vi "Filter Dialog.vi"() -> (0 "error out":errorcluster, 2 "Base Filter out":refnum<class "Base Filter.lvclass">, 3 "Valid Filter Configuration":bool)   [LabVIEW 2018, in "Assert API Components.lvlib" / "Assert Display.lvlib" / "Filter Config Display.lvlib" / "Filter Config Display.lvclass"]
doc: "Filter definition window - allows the user to create new filters on the fly to display/not display assert values in the UI"
uses:
  Filter Config Display.lvclass
  Assert API Components/Filter Type.ctl
  Assert API Components/Filter By Time.ctl
  Assert API Components/Filter By String.ctl
  Assert API Components/Filter Configurations/Base Filter.lvclass
  Assert API Components/Boolean Filter Configuration.ctl
  Assert API Components/Time Filter Configuration.ctl
  Assert API Components/String Filter Configuration.ctl
  Assert API Components/Filter Configurations/Base Filter.lvclass/Base Filter.ctl
  <vilib>/Utility/config.llb/Read Key (String).vi
  Assert Display/Assert Display.lvlib
  Assert API Components/Assert API Components.lvlib
  <vilib>/Utility/config.llb/NI_LVConfig.lvlib
panel:
  in  "Tab Control":enum32{"Boolean", "String", "Time"}(tab)
  in  "Status":bool
  in  "Filter String":T1
  in  "String Comparison Method":T2(ring)
  in  "Filter Value":string
  in  "Filter Time":T3
  in  "Time Comparison Method":enum16{"Before", "After"}(ring)
  in  "Filter Timestamp":timestamp
  in  "Include or Exclude":enum16{"Include", "Exclude"}(ring)
  in  "Filter Type":T4
  in  "OK Button":bool
  in  "Description":string
  in  "Filter Name":string
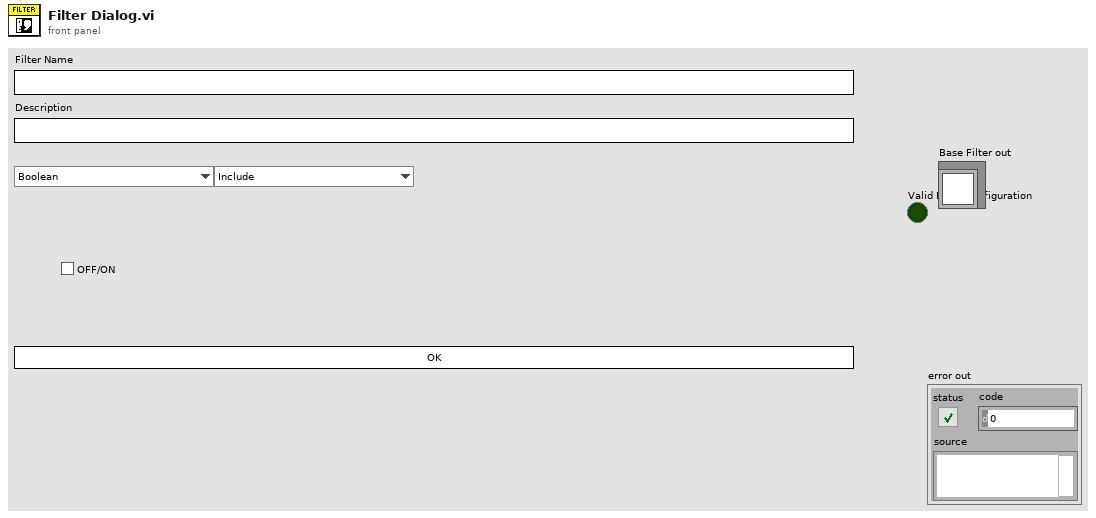
[diagram p1: front panel]
types:
  T1 = typedef "Assert API Components.lvlib/Assert Display.lvlib/Filter By String.ctl" = enum16{"Assert Builder User Name", "Assert Name", "Assert VI Name", "Calling VI Name", "Comment", "Data Type", "Evaluation String"}
  T2 = enum16{"Contains", "Does Not Contain", "Starts With", "Equals", "Does Not Equal"}
  T3 = typedef "Assert API Components.lvlib/Assert Display.lvlib/Filter By Time.ctl" = enum16{"Assert Build Timestamp", "Last Update Timestamp"}
  T4 = typedef "Assert API Components.lvlib/Assert Display.lvlib/Filter Type.ctl" = enum16{"Boolean", "String", "Time"}
  T5 = typedef "Assert API Components.lvlib/Assert Display.lvlib/String Filter Configuration.ctl" = cluster{"Filter String":T1, "String Comparison Method":enum16{"Contains", "Does Not Contain", "Starts With", "Equals", "Does Not Equal"}, "Comparison Value":string}
  T6 = typedef "Assert API Components.lvlib/Assert Display.lvlib/Time Filter Configuration.ctl" = cluster{"Filter Time":T3, "Time Comparison Method":enum16{"Before", "After"}, "Time Stamp":timestamp}
  T7 = typedef "Assert API Components.lvlib/Assert Display.lvlib/Boolean Filter Configuration.ctl" = cluster{"Boolean Comparison Value":bool}
  T8 = typedef "NI_LVConfig.lvlib/Config Data RefNum.ctl" = refnum<k1>
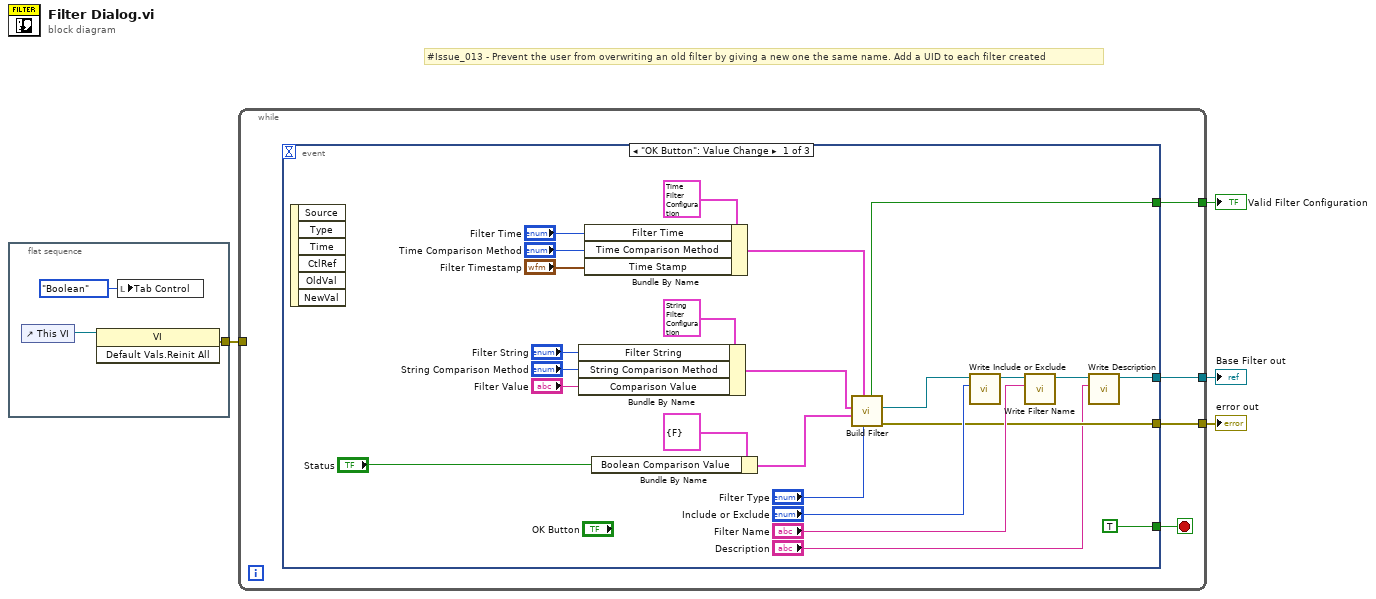
[diagram p0: block diagram]
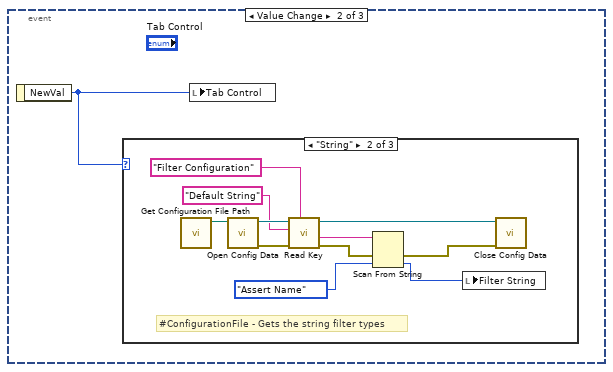
[diagram p2: hidden frame]
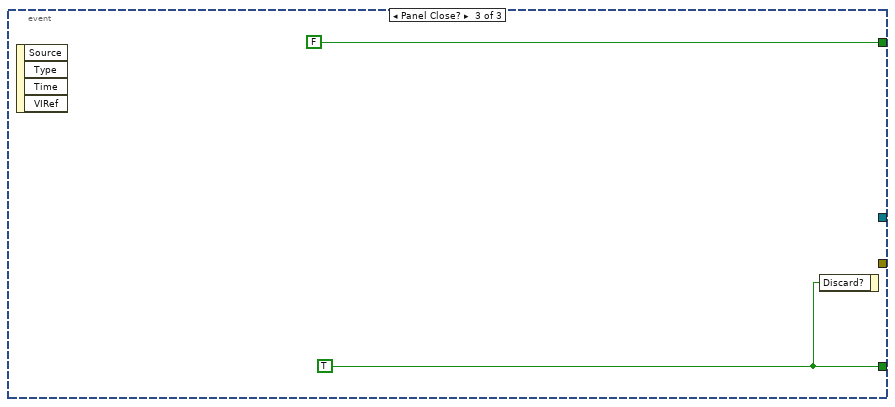
[diagram p5: hidden frame]
diagram:
  # "#Issue_013 - Prevent the user from overwriting an old filter by giving a new one the same name. Add a UID to each filter created"
  n1 = flat-sequence {
    tunnel: [w5] -> w1
    frame #0 {
      n2 = control-ref of="This VI"() -> (w6:refnum<vi>)
      n3 = invoke class="VI" method="Default Vals.Reinit All"(reference=w6) -> (error out=w5:errorcluster)  [unwired: 2 in, 2 out]
      n4 = local write "Tab Control"(enum32{"Boolean", "String", "Time"}."Boolean" ("Tab Control")) -> ()
    }
  }
  n5 = while {
    tunnel: [w10] -> w4
    tunnel: [w9] -> w3
    tunnel: [w8] -> w2
    tunnel: w1 -> [_]
    stop <- w11 stop-if-true
    n6 = event shown="[0] \"OK Button\": Value Change" {
      selector: _ -> [_ _ _]
      dyn-events: _ -> [_ _ _]
      timeout: _ -> [_ _ _]
      tunnel: [TRUE _ w49] -> w11
      tunnel: [w21 _ FALSE] -> w10
      tunnel: [w13 _ _] -> w9
      tunnel: [w14 _ _] -> w8
      event "OK Button": Value Change {
        n7 = event-data() -> ()  [unwired: 1 in, 6 out]
        n8 = Bundle By Name(cluster=T5 {"Filter String"=enum."Assert Builder User Name", "String Comparison Method"=enum."Contains", "Comparison Value"=""}, "Filter String"="Filter String", "String Comparison Method"="String Comparison Method", "Comparison Value"="Filter Value") -> (w29:T5)
        n9 = Bundle By Name(cluster=T6 {"Filter Time"=enum."Assert Build Timestamp", "Time Comparison Method"=enum."Before", "Time Stamp"=timestamp(0 s since 1904-01-01)}, "Filter Time"="Filter Time", "Time Comparison Method"="Time Comparison Method", "Time Stamp"="Filter Timestamp") -> (w27:T6)
        n10 = Bundle By Name(cluster=T7 {"Boolean Comparison Value"=FALSE}, "Boolean Comparison Value"="Status") -> (w28:T7)
        n11 = call "Build Filter.vi"("Filter Type"="Filter Type", "Time Filter Configuration"=w27, "Boolean Filter Configuration"=w28, "String Filter Configuration"=w29) -> ("error out"=w14:errorcluster, "Base Filter out"=w31:refnum<class "Base Filter.lvclass">, "Boolean"=w21:bool)  [unwired: 5 in]
        n12 = call "Write Include or Exclude.vi"("Include or Exclude"="Include or Exclude", "Base Filter in"=w31) -> ("Base Filter out"=w34:refnum<class "Base Filter.lvclass">)  [unwired: 9 in]
        n13 = call "Write Filter Name.vi"("Filter Name"="Filter Name", "Base Filter in"=w34) -> ("Base Filter out"=w15:refnum<class "Base Filter.lvclass">)  [unwired: 9 in]
        n14 = call "Write Description.vi"("Description"="Description", "Base Filter in"=w15) -> ("Base Filter out"=w13:refnum<class "Base Filter.lvclass">)  [unwired: 9 in]
      }
      event Value Change {
        n15 = event-data() -> ("NewVal"=w36:T4)  [unwired: 1 in]
        n16 = case shown="\"String\"" w36 {
          frame "Boolean", Default {
          }
          frame "String" {
            # "#ConfigurationFile - Gets the string filter types"
            n17 = call "Get Configuration File Path.vi"() -> ("Configuration File Path"=w47:path)  [unwired: 11 in]
            n18 = call <vilib>:"Open Config Data.vi"("configuration file path"=w47) -> ("error out"=w45:errorcluster, "refnum"=w46:T8)  [unwired: 8 in, 1 out]
            n19 = call-poly <vilib>:"Read Key.vi"("section"="Filter Configuration", "error in (no error)"=w45, "key"="Default String", "refnum"=w46) -> ("error out"=w41:errorcluster, "value"=w38:string, "refnum out"=w44:T8)  [unwired: 4 in, 1 out]
            n20 = Scan From String(input string=w38, error in=w41, default 1=Filter_By_String."Assert Name" ("Filter String")) -> (error out=w40:errorcluster, output 1=w37:T1)  [unwired: 2 in, 2 out]
            n21 = local write "Filter String"(w37) -> ()
            n22 = call <vilib>:"Close Config Data.vi"("error in (no error)"=w40, "refnum"=w44) -> ()  [unwired: 8 in, 2 out]
          }
          frame "Time" {
          }
        }
        n23 = local write "Tab Control"(w36) -> ()
      }
      event Panel Close? {
        w49 = TRUE
        n24 = event-data() -> ()  [unwired: 1 in, 4 out]
        n25 = event-data("Discard?"=w49) -> ()  [unwired: 1 in, 1 out]
      }
    }
  }
  "Valid Filter Configuration" <- w4
  "Base Filter out" <- w3
  "error out" <- w2
